vi "Ensure Error Logs Folder Is Valid.vi"(8 "Error In":errorcluster, 10 "Application Name":string, 11 "Error Logs Folder (as provided by calling application)":path) -> (0 "Error Out":errorcluster, 3 "Error Logs Folder (valid)":path)   [LabVIEW 2016, in "Error Manager.lvlib"]
doc: "This VI checks that the Error Logs Folder path is valid, and that it points to an existing folder. If it does, this VI simply passes that input to the output. If it doesn't, this VI:\n1. Replaces the folder path provided with an automatically generated folder path\n2. Displays a one-button dialogue that informs the user"
uses:
  Error Manager.lvlib
  <vilib>/Utility/sysdir.llb/System Directory Type.ctl
panel:
  # "Development\nControls or indicators that are useful for development or testing, but which are not outputs of the VI."
  # "Input\nInputs to the VI"
  # "Output\nOutputs of the VI"
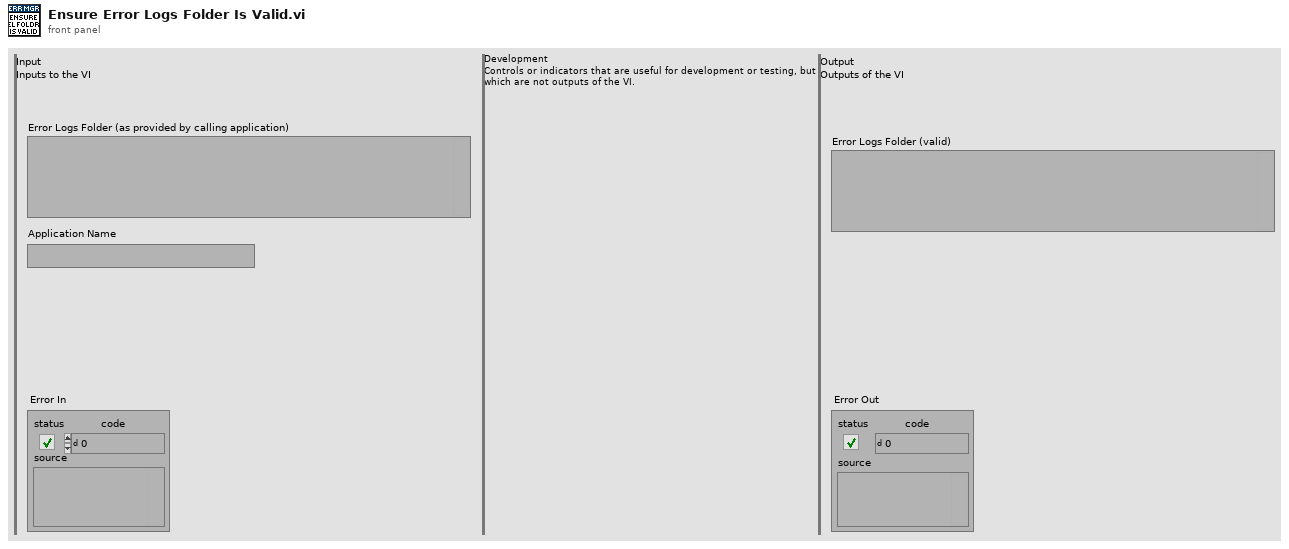
[diagram p1: front panel]
types:
  T1 = typedef "System Directory Type.ctl" = i32
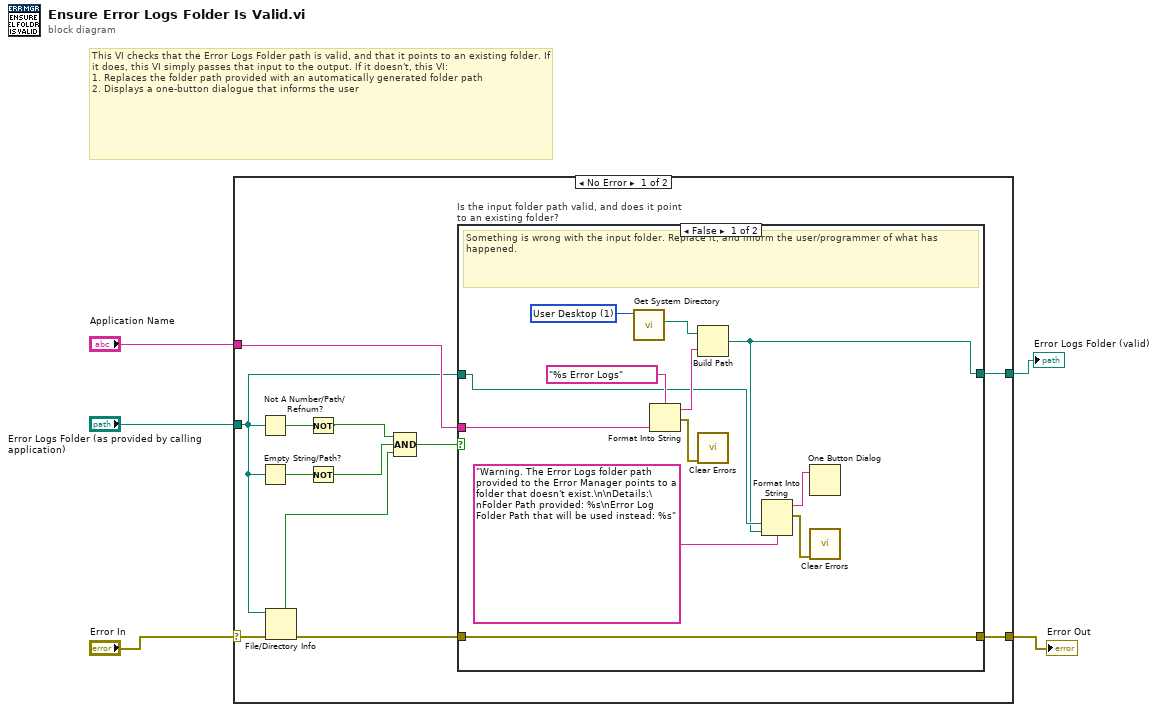
[diagram p0: block diagram]
diagram:
  # "This VI checks that the Error Logs Folder path is valid, and that it points to an existing folder. If it does, this VI simply passes that input to the output. If it doesn't, this VI:\n1. Replaces the folder path provided with an automatically generated folder path\n2. Displays a one-button dialogue that informs the user"
  n1 = case shown="No Error" "Error In" {
    selector: "Error In" -> [w17 w32]
    tunnel: [w10 w32] -> w4
    tunnel: "Error Logs Folder (as provided by calling application)" -> [w7 _]
    tunnel: "Application Name" -> [w8 _]
    tunnel: [w6 _] -> w1
    frame No Error {
      n2 = Not A Number/Path/Refnum?(number/path/refnum=w7) -> (NaN/Path/Refnum?=w15:bool)
      n3 = Empty String/Path?(string/path=w7) -> (empty?=w14:bool)
      n4 = File/Directory Info(path=w7, error in=w17) -> (directory=w11:bool, error out=w16:errorcluster)  [unwired: 5 out]
      n5 = Not(x=w15) -> (.not. x?=w13:bool)
      n6 = Not(x=w14) -> (.not. x?=w12:bool)
      n7 = Compound Arithmetic op=AND(w13, w12, w11) -> (w9:bool)
      n8 = case "Is the input folder path valid, and does it point to an existing folder?" shown="False" w9 {
        tunnel: w16 -> [w28 w31]
        tunnel: [w28 w31] -> w10
        tunnel: w8 -> [w23 _]
        tunnel: w7 -> [w19 w30]
        tunnel: [w18 w30] -> w6
        frame False {
          w29 = T1 1 items=["User Home"=0, "User Desktop"=1, "User Documents"=2, "User Application Data"=3, "User Preferences"=4, "User Temporary"=5, "Public Documents"=6, "Public Application Data"=7, "Public Preferences"=8, "Public Cache"=13, "System Core Libraries"=9, "System Installed Libraries"=10, "Application Files"=11, "Boot Volume Root"=12] ("system directory type")
          # "Something is wrong with the input folder. Replace it, and inform the user/programmer of what has happened."
          n9 = call <vilib>:"Get System Directory.vi"("system directory type"=w29) -> ("system directory"=w27:path)  [unwired: 10 in]
          n10 = Format Into String(format string="%s Error Logs", w23) -> (resulting string=w25:string, error out=w24:errorcluster)  [unwired: 2 in]
          n11 = Build Path(base path=w27, name or relative path=w25) -> (appended path=w18:path)
          n12 = call <vilib>:"Clear Errors.vi"("error in (no error)"=w24) -> ()  [unwired: 5 in, 2 out]
          n13 = Format Into String(format string="Warning. The Error Logs folder path provided to the Error Manager points to a folder that doesn't exist.\n\nDetails:\nFolder Path provided: %s\nError Log Folder Path that will be used instead: %s", w19, w18) -> (resulting string=w20:string, error out=w22:errorcluster)  [unwired: 2 in]
          n14 = One Button Dialog(message=w20) -> ()  [unwired: 1 in, 1 out]
          n15 = call <vilib>:"Clear Errors.vi"("error in (no error)"=w22) -> ()  [unwired: 5 in, 2 out]
        }
        frame True {
          # "The input folder is all good. Use it."
        }
      }
    }
    frame Error {
    }
  }
  "Error Out" <- w4
  "Error Logs Folder (valid)" <- w1
